vi "Display_Console.vi"(8 "error in":errorcluster) -> (0 "error out":errorcluster)   [LabVIEW 2013, in "Display Console.lvlib"]
doc: "This is the top level of the simulated console module (a free running module of the ATM simulator). \n\nIt is closed using a user event. It communicates with the other modules using a queue based API which has comms modules that can be swapped if required. \n\n[Covers: UI3]"
uses:
  Display Console.lvlib
  User Events/Controls/UE Abort Action.ctl
  Private Controls/Display Action.ctl
  Private Controls/Module Data Cluster.ctl
  Error Handler/Error Handler.lvlib
  Private Controls/Display_Data.ctl
panel:
  out "Card Read":bool
  out "Message Screen":string
  out "Current Transaction":string
  # "[Covers: UI1]"
  # "[Covers: UI3B]"
  # "[Covers: UI3C]"
  # "[Covers: UI3A]"
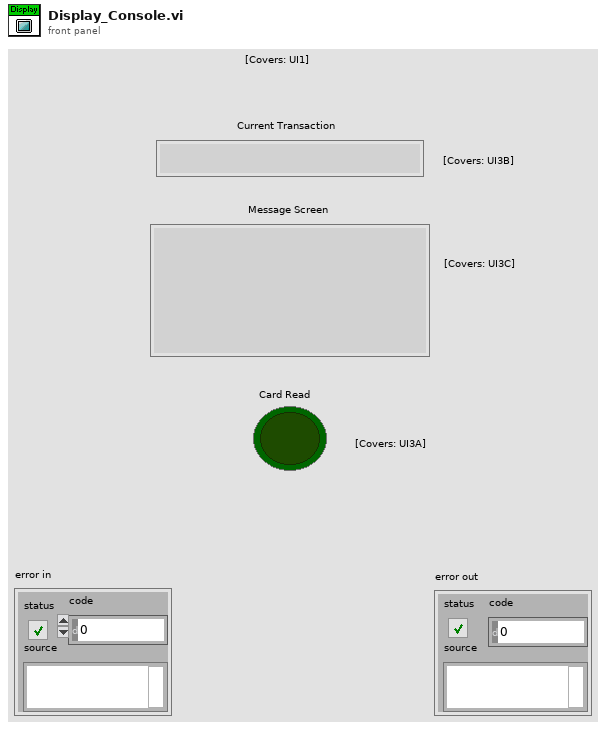
[diagram p1: front panel]
types:
  T1 = typedef "Display Console.lvlib/Display_Data.ctl" = cluster{"Current Transaction":string, "Message Screen":string, "Card Read":bool}
  T2 = typedef "Display Console.lvlib/Module Data Cluster.ctl" = cluster{"Data":variant, "Action":T3}
  T3 = typedef "Display Console.lvlib/Display Action.ctl" = enum16{"Init", "Message", "Transaction", "Card", "Exit", "Error"}
  T4 = typedef "UE Abort Action.ctl" = enum16{"Destroy", "Get", "Create"}
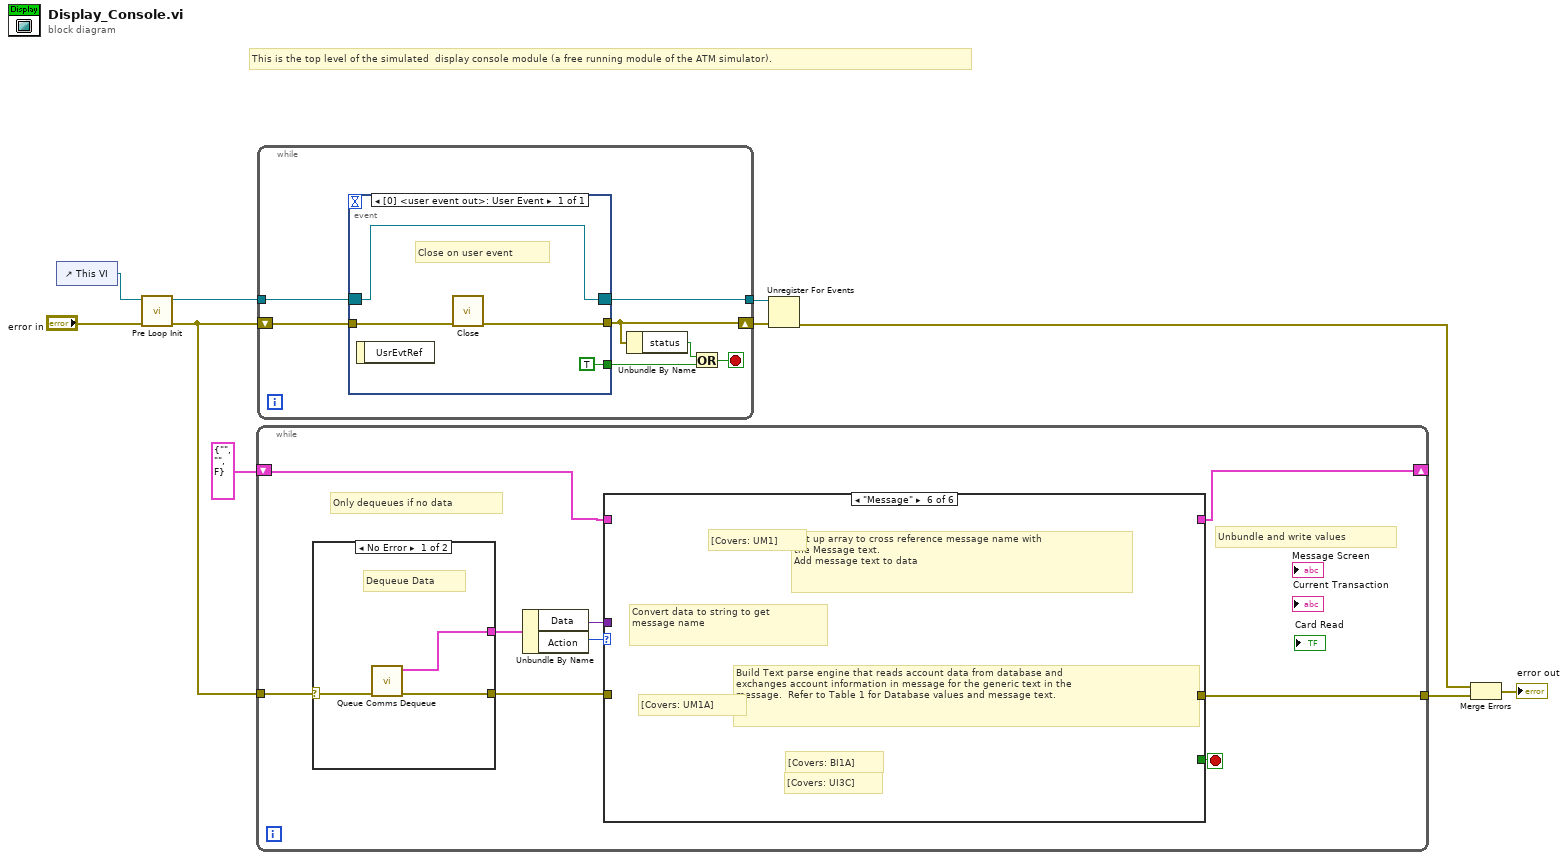
[diagram p0: block diagram]
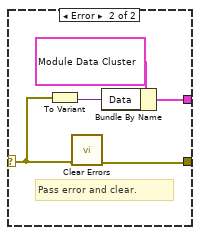
[diagram p2: hidden frame]
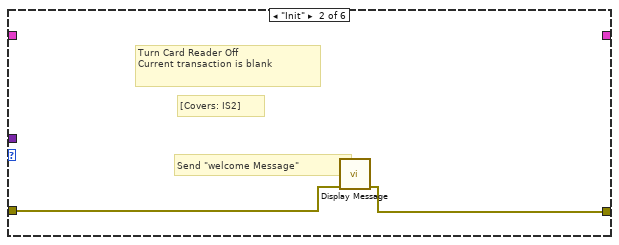
[diagram p4: hidden frame]
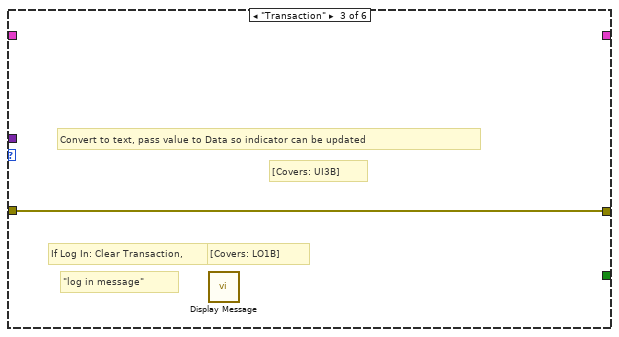
[diagram p5: hidden frame]
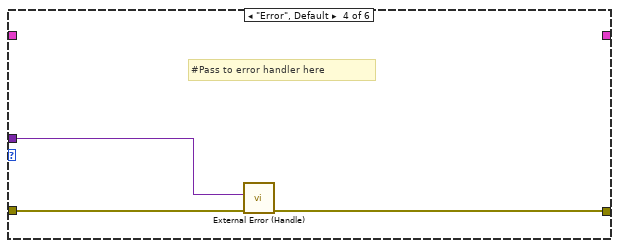
[diagram p6: hidden frame]
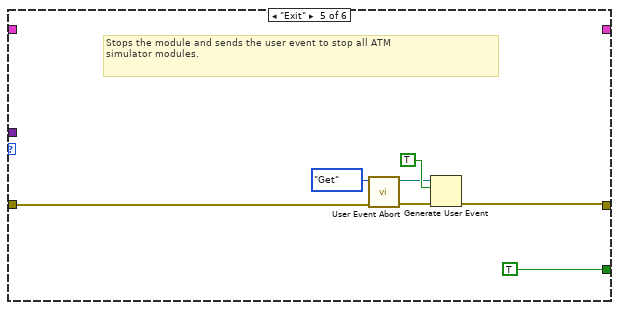
[diagram p7: hidden frame]
diagram:
  # "This is the top level of the simulated  display console module (a free running module of the ATM simulator)."
  n1 = control-ref of="This VI"() -> (w10:refnum<vi>)
  n2 = call "Pre Loop Init.vi"("error in"="error in", "Ref In"=w10) -> ("error out"=w5:errorcluster, "Event Registration Refnum"=w8:refnum<event-registration>)  [unwired: 8 in]
  n3 = while {
    tunnel: w5 -> [w18]
    tunnel: [w13] -> w3
    shift-right: [w11] -> _
    shift-left: T1 {"Current Transaction"="", "Message Screen"="", "Card Read"=FALSE} ("Display Data") -> [w12]
    stop <- w19 stop-if-true
    # "Unbundle and write values"
    # "Only dequeues if no data"
    n4 = case shown="No Error" w18 {
      selector: w18 -> [w21 w24]
      tunnel: [w22 w23] -> w16
      tunnel: [w20 w25] -> w17
      frame No Error {
        # "Dequeue Data"
        n5 = call "Queue Comms Dequeue.vi"("error in"=w21) -> ("error out"=w22:errorcluster, "Data Out"=w20:T2)  [unwired: 9 in]
      }
      frame Error {
        # "Pass error and clear."
        n6 = To Variant(anything=w24) -> (Variant=w26:variant)
        n7 = call <vilib>:"Clear Errors.vi"("error in (no error)"=w24) -> ("error out"=w23:errorcluster)  [unwired: 6 in]
        n8 = Bundle By Name(cluster=T2 {"Data"=variant, "Action"=enum."Transaction"} ("Cluster"), "Data"=w26) -> (w25:T2)
      }
    }
    n9 = Unbundle By Name(w17) -> ("Data"=w14:variant, "Action"=w15:T3)
    n10 = case shown="\"Message\"" w15 {
      tunnel: [_ _ _ _ TRUE _] -> w19
      tunnel: w16 -> [w29 w31 w32 w35 w37 _]
      tunnel: w14 -> [_ _ _ w33 _ _]
      tunnel: [w29 w30 w32 w34 w36 _] -> w13
      tunnel: w12 -> [w28 _ _ _ _ _]
      tunnel: [w28 _ _ _ _ _] -> w11
      frame "Card" {
        # "[Covers: UI3A]"
        # "[Covers: L01B]"
        # "No conversion required, \none intent message"
        # "Turn card Indicator ON by Adding new value to Data"
      }
      frame "Init" {
        # "Send \"welcome Message\""
        # "[Covers: IS2]"
        # "Turn Card Reader Off\nCurrent transaction is blank"
        n11 = call "Display Message.vi"("error in"=w31) -> ("error out"=w30:errorcluster)  [unwired: 10 in]
      }
      frame "Transaction" {
        # "[Covers: LO1B]"
        # "\"log in message\""
        # "If Log In: Clear Transaction,"
        # "[Covers: UI3B]"
        # "Convert to text, pass value to Data so indicator can be updated"
        n12 = call "Display Message.vi"() -> ()  [unwired: 11 in, 1 out]
      }
      frame "Error", Default {
        # "#Pass to error handler here"
        n13 = call "External Error (Handle).vi"("error in"=w35, "Data"=w33) -> ("error out"=w34:errorcluster)  [unwired: 9 in]
      }
      frame "Exit" {
        # "Stops the module and sends the user event to stop all ATM\nsimulator modules."
        n14 = call "User Event Abort.vi"("error in"=w37, "Action"=UE_Abort_Action."Get") -> ("error out"=w39:errorcluster, "user event out"=w40:refnum<user-event>)  [unwired: 8 in]
        n15 = Generate User Event(user event=w40, event data cluster=TRUE ("event data"), error in=w39) -> (error out=w36:errorcluster)  [unwired: 1 in, 1 out]
      }
      frame "Message" {
        # "[Covers: BI1A]"
        # "[Covers: UI3C]"
        # "[Covers: UM1A]"
        # "Build Text parse engine that reads account data from database and\nexchanges account information in message for the generic text in the \nmessage.  Refer to Table 1 for Database values and message text."
        # "[Covers: UM1]"
        # "Convert data to string to get \nmessage name"
        # "Set up array to cross reference message name with\nthe Message text.\nAdd message text to data"
      }
    }
  }
  n16 = while {
    shift-right: [w46] -> w7
    shift-left: w5 -> [w49]
    tunnel: w8 -> [w44]
    tunnel: [w43] -> w6
    stop <- w47 stop-if-true
    n17 = event shown="[0] <user event out>: User Event" {
      selector: w44 -> [w53]
      dyn-events: [w53] -> w43
      timeout: _ -> [_]
      tunnel: w49 -> [w52]
      tunnel: [w51] -> w46
      tunnel: [TRUE ("stop")] -> w48
      event User Event {
        # "Close on user event"
        n18 = event-data() -> ()  [unwired: 1 in, 1 out]
        n19 = call "Close.vi"("error in"=w52) -> ("error out"=w51:errorcluster)  [unwired: 10 in]
      }
    }
    n20 = Unbundle By Name(w46) -> ("status"=w45:bool)
    n21 = Or(x=w45, y=w48) -> (x .or. y?=w47:bool)
  }
  n22 = Unregister For Events(event registration refnum=w6, error in=w7) -> (error out=w2:errorcluster)
  n23 = Merge Errors(w2, w3) -> (→"error out":errorcluster)
